vi "CAN COMMS.vi"() -> ()   [LabVIEW 2022 SP3]
uses:
  <vilib>/xnet/xnet.llb/XNET Frame CAN.ctl
  <vilib>/xnet/xnet.llb/XNET Frame Type CAN.ctl
  <vilib>/xnet/xnet.llb/XNET Create Session (Frame Input Stream).vi
  <vilib>/xnet/xnet.llb/XNET Create Session (Frame Output Queued).vi
  <vilib>/xnet/xnet.llb/XNET Write (Frame CAN).vi
  <vilib>/xnet/xnet.llb/XNET Read (Frame CAN).vi
  <resource>/objmgr/xnet.rc
panel:
  in  "Interface:CAN:Termination":u32(ring) items=["Off", "On"]
  out "data 2":T1[](array[typedef]) {"payload" format="%x"; "timestamp" format="%<%.7X\n%x>T"; "type" items=["CAN Data"=0, "CAN Remote"=1, "CAN Bus Error"=2, "CAN 2.0 Data"=8, "CAN FD Data"=16, "CAN FD+BRS Data"=24, "J1939 Data"=192, "Delay"=224, "Log Trigger"=225, "Start Trigger"=226]; "identifier" format="%x"}
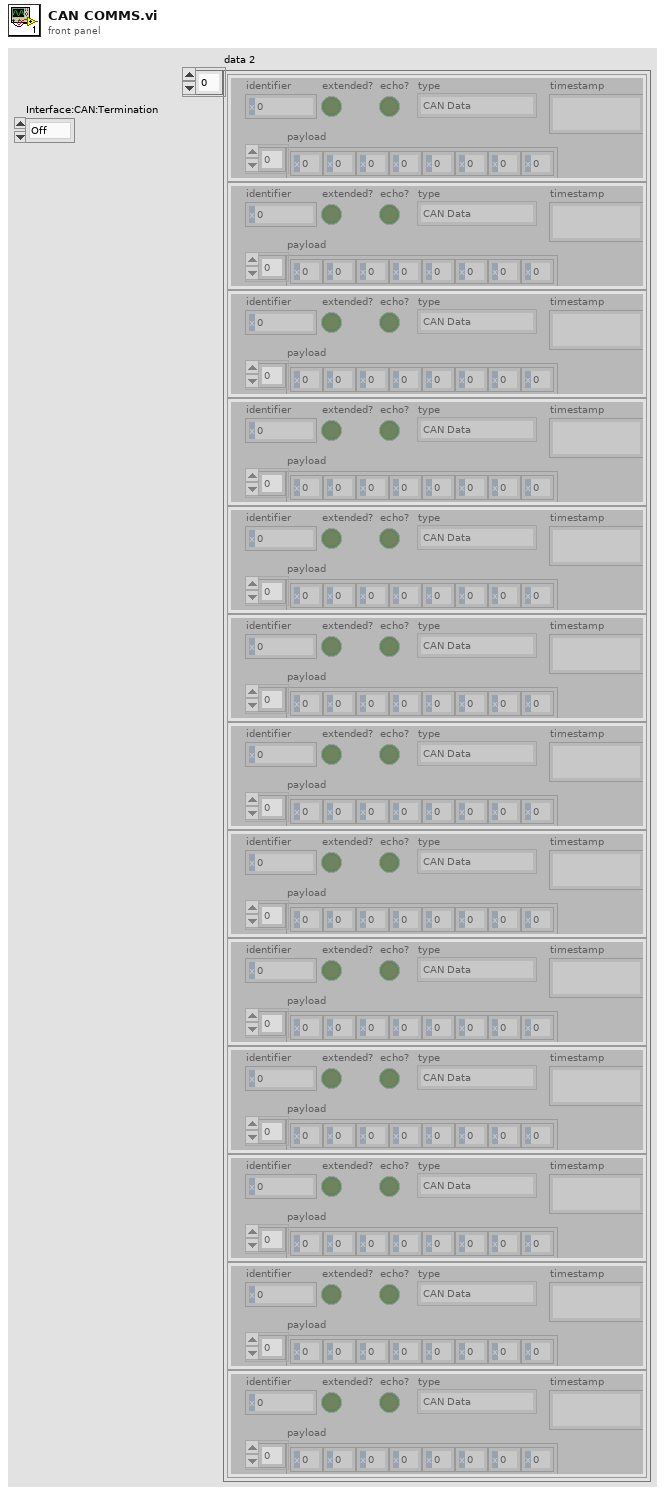
[diagram p1: front panel]
types:
  T1 = typedef "XNET Frame CAN.ctl" = cluster{"timestamp":timestamp, "payload":u8[], "identifier":u32, "type":T2, "extended?":bool, "echo?":bool}
  T2 = typedef "XNET Frame Type CAN.ctl" = u8
  T3 = cluster{"data[0]":T1, "data[1]":T1, "data[2]":T1, "data[3]":T1, "data[4]":T1, "data[5]":T1, "data[6]":T1, "data[7]":T1, "data[8]":T1}
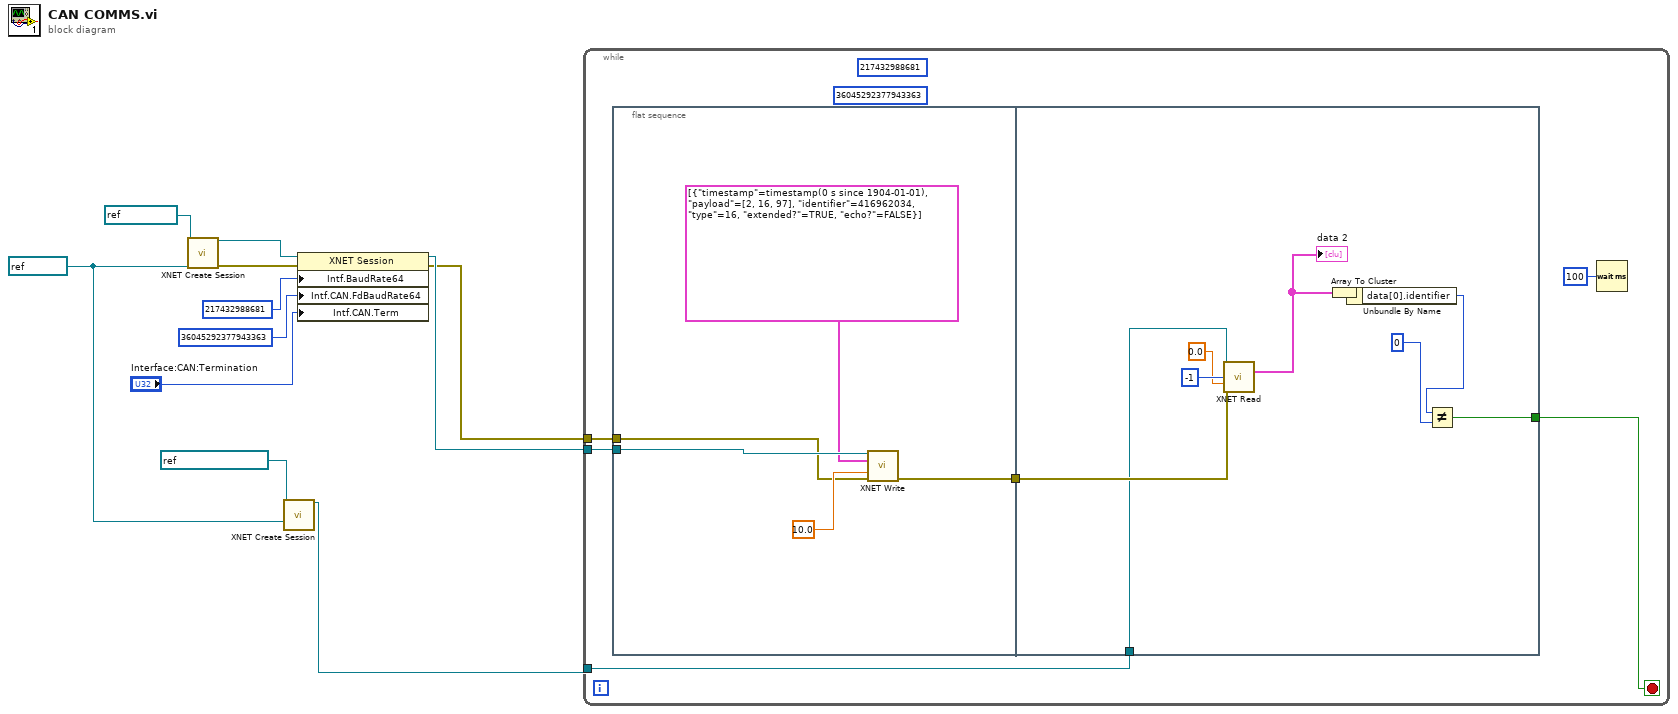
[diagram p0: block diagram]
diagram:
  w4 = refnum<k21> "CAN1" ("interface")
  n1 = call-poly <vilib>:"XNET Create Session.vi"("frame"=refnum<k21> "Escritura\nElatch_Labview", "interface"=w4) -> ("session out"=w11:refnum<k21>, "error out"=w10:errorcluster)  [unwired: 12 in]
  n2 = call-poly <vilib>:"XNET Create Session.vi"("cluster (:memory:)"=refnum<k21> "Elatch_Labview", "interface"=w4) -> ("session out"=w6:refnum<k21>)  [unwired: 12 in, 1 out]
  n3 = property class="XNET Session"(reference=w11, error in=w10, "Intf.BaudRate64"=u64 217432988681 ("Interface:64bit Baud Rate"), "Intf.CAN.FdBaudRate64"=u64 36045292377943363 ("Interface:CAN:64bit FD Baud Rate"), "Intf.CAN.Term"="Interface:CAN:Termination") -> (reference out=w2:refnum<k21>, error out=w1:errorcluster)
  n4 = while {
    tunnel: w6 -> [w13]
    tunnel: w2 -> [w17]
    tunnel: w1 -> [w16]
    stop <- w15 stop-if-true
    (unwired) u64 36045292377943363 ("Interface:CAN:64bit FD Baud Rate")
    (unwired) u64 217432988681 ("Interface:64bit Baud Rate")
    n5 = flat-sequence {
      tunnel: w17 -> [w22]
      tunnel: w16 -> [w19]
      tunnel: [w18] -> w14
      tunnel: [w25] -> w15
      tunnel: w14 -> [w24]
      tunnel: w13 -> [w23]
      frame #0 {
        n6 = call-poly <vilib>:"XNET Write.vi"("session in"=w22, "data"=T1[] [{"timestamp"=timestamp(0 s since 1904-01-01), "payload"=[2, 16, 97], "identifier"=416962034, "type"=16, "extended?"=TRUE, "echo?"=FALSE}], "timeout (10)"=10.0, "error in (no error)"=w19) -> ("error out"=w18:errorcluster)  [unwired: 10 in, 1 out]
      }
      frame #1 {
        n7 = call-poly <vilib>:"XNET Read.vi"("session in"=w23, "number to read (-1)"=-1, "timeout (0)"=0.0, "error in (no error)"=w24) -> ("data"=w30:T1[])  [unwired: 8 in, 3 out]
        "data 2" <- w30
        n8 = Array To Cluster(array=w30) -> (cluster=w31:T3)
        n9 = Unbundle By Name(w31) -> ("data[0].identifier"=w26:u32)
        n10 = Not Equal?(x=w26, y=u32 0) -> (x != y?=w25:bool)
      }
    }
    n11 = Wait (ms)(milliseconds to wait=u32 100) -> ()  [unwired: 1 out]
  }
